vi "_SN&SNNum_vna_wmg.vi"(1 "SNNum":string, 2 "SN":string) -> (0 "SN_out":string)   [LabVIEW 2011]
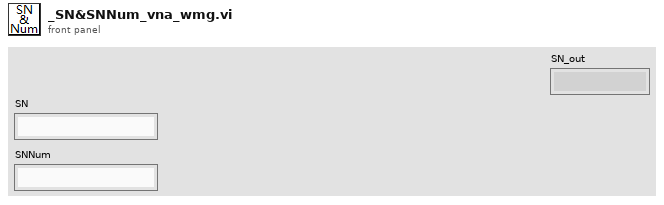
[diagram p1: front panel]
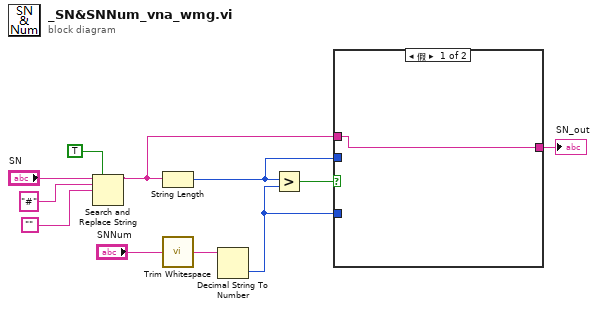
[diagram p0: block diagram]
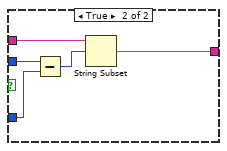
[diagram p2: hidden frame]
diagram:
  n1 = Search and Replace String(replace all?=TRUE ("替换全部？(F)"), input string="SN", search string="#" ("搜索字符串"), replace string="") -> (result string=w3:string)  [unwired: 4 in, 3 out]
  n2 = String Length(string=w3) -> (length=w8:i32)
  n3 = call <vilib>:"Trim Whitespace.vi"("string"="SNNum") -> ("trimmed string"=w10:string)  [unwired: 1 in]
  n4 = Decimal String To Number(string=w10) -> (number=w7:i32)  [unwired: 2 in, 1 out]
  n5 = Greater?(x=w8, y=w7) -> (0:w9:bool)
  n6 = case shown="假" w9 {
    tunnel: w3 -> [w12 w15]
    tunnel: w8 -> [_ w17]
    tunnel: w7 -> [_ w16]
    tunnel: [w12 w13] -> w1
    frame False {
    }
    frame True {
      n7 = Subtract(x=w17, y=w16) -> (x-y=w14:i32)
      n8 = String Subset(string=w15, offset (0)=w14) -> (substring=w13:string)  [unwired: 1 in]
    }
  }
  "SN_out" <- w1
